vi "API String - Set Float Precision.vi"(8 "Error in":errorcluster caption="Error in (no error)", 11 "Precision":u8) -> (0 "Error out":errorcluster)   [LabVIEW 2017, in "API String Arguments Support.lvlib"]
uses:
  API String Arguments Support.lvlib
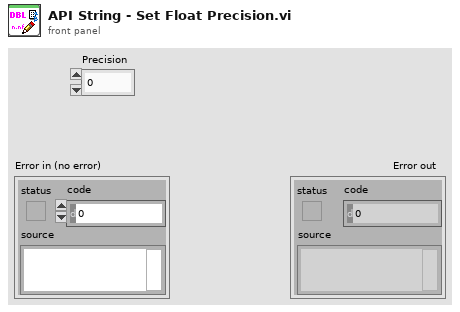
[diagram p1: front panel]
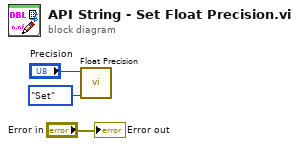
[diagram p0: block diagram]
diagram:
  n1 = call "Float Precision.vi"("Enum"=enum16{"Set", "Get"}."Set", "Precision"="Precision") -> ()  [unwired: 8 in, 2 out]
  "Error out" <- "Error in"
